vi "根据旋转角度计算螺丝刀中心偏移量.vi"(9 "上视觉：螺丝与Gold影像需要补偿角度":dbl, 11 "dtx,dty In":T2) -> (3 "dtx,dty Out":T2)   [LabVIEW 2014]
uses:
  Global.vi
  Controls/XYZPos.ctl
  Controls/XYPos.ctl
panel:
  out "机械手需要转多少度才能将刀和槽对准":dbl
  out "下视觉：螺丝刀与Gold影像需要补偿角度":dbl
  in  "下视觉：螺丝刀回原点后角度":dbl
  in  "下视觉：Gold影像角度":dbl
  in  "1":T1 {"X" format="%#.3f"}
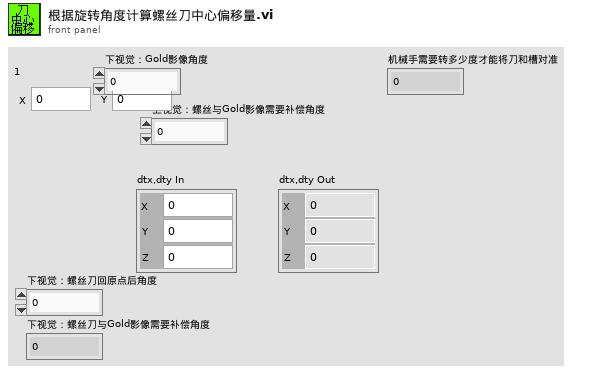
[diagram p1: front panel]
types:
  T1 = typedef "XYPos.ctl" = cluster{"X":dbl, "Y":dbl}
  T2 = typedef "XYZPos.ctl" = cluster{"X":dbl, "Y":dbl, "Z":dbl}
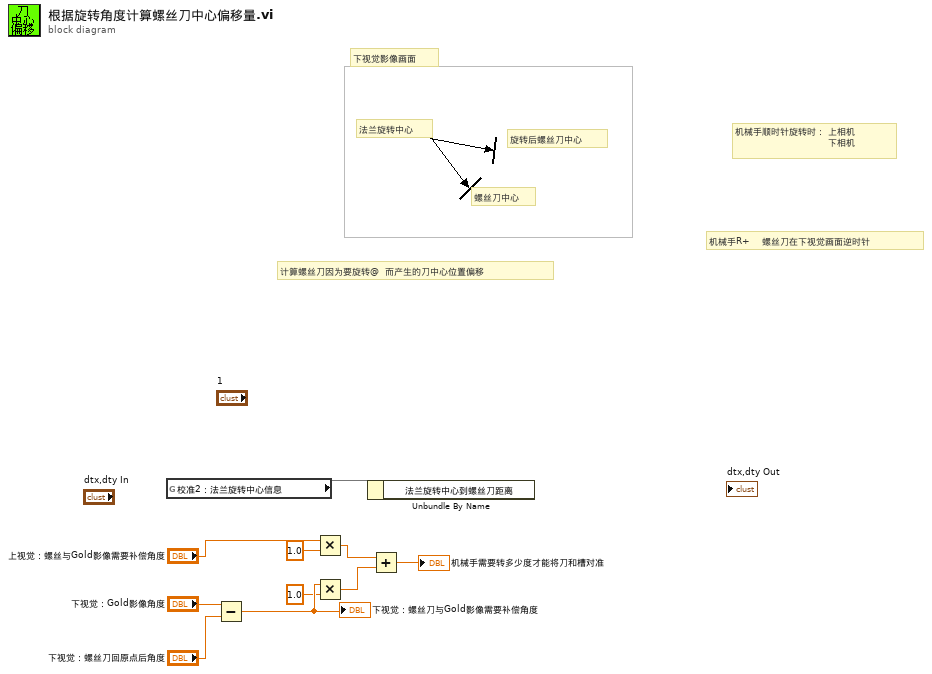
[diagram p0: block diagram]
diagram:
  # "机械手R+    螺丝刀在下视觉画面逆时针"
  # "机械手顺时针旋转时： 上相机\n                               下相机"
  # "旋转后螺丝刀中心"
  # "螺丝刀中心"
  # "法兰旋转中心"
  # "下视觉影像画面"
  # "计算螺丝刀因为要旋转@  而产生的刀中心位置偏移"
  n1 = global read "Global.vi" "校准2：法兰旋转中心信息"() -> (w10)
  n2 = Subtract(x="下视觉：Gold影像角度", y="下视觉：螺丝刀回原点后角度") -> (x-y=w5:dbl)
  "下视觉：螺丝刀与Gold影像需要补偿角度" <- w5
  n3 = Multiply(x="上视觉：螺丝与Gold影像需要补偿角度", y=1.0) -> (x*y=w3:dbl)
  n4 = Multiply(x=w5, y=1.0) -> (x*y=w2:dbl)
  n5 = Unbundle By Name(w10) -> ()  [unwired: 1 out]
  n6 = Add(x=w3, y=w2) -> (x+y=→"机械手需要转多少度才能将刀和槽对准":dbl)
